vi "Finish.vi"   [LabVIEW 2015]
doc: "This VI is called just before exiting. It is expected to close I/O refnum, save collected data, etc."
uses:
  <vilib>/Rock Robotics/WPI/Utilities/WPI_GetSetVariantRefNum.vi
  <vilib>/Rock Robotics/WPI/Ultrasonic/WPI_SonarMB1010DigitalRefNum Registry Get.vi
  <vilib>/Rock Robotics/WPI/Ultrasonic/WPI_SonarMB1010DigitalClose.vi
types:
  T1 = typedef "WPI_SonarMB1010DigitalDeviceRef.ctl" = cluster{"CounterDevRef":T2, "Scaling factor (s/in)":dbl}
  T2 = typedef "WPI_CounterDevRef.ctl" = cluster{"DevStatus":errorcluster, "CntIndex":T3}
  T3 = typedef "FPGA_CounterCtrSystemIndex.ctl" = enum8{"Ctr 0", "Ctr 1", "Ctr 2", "Ctr 3", "Ctr 4", "Ctr 5", "Ctr 6", "Ctr 7", "Invalid"}
  T4 = typedef "WPI_JoystickDevRef.ctl" = cluster{"Device":T5}
  T5 = typedef "WPI_JoystickDeviceEnum.ctl" = enum16{"USB 0", "USB 1", "USB 2", "USB 3", "USB 4", "USB 5"}
  T6 = typedef "WPI_MotorControlDeviceRef.ctl" = cluster{"DeviceStatus":errorcluster, "Type":T7, "PWM":cluster{"PWM Channel":T8, "DeadBand":T9}, "CAN":cluster{"Device Number":u8, "Control Mode":T10, "Semaphore":T11, "Max Vout":dbl, "TalonSRX Control Mode":T12}, "Invert":bool}
  T7 = typedef "WPI_MotorControlType.ctl" = enum16{"PWM", "CAN", "CANTalonSRX"}
  T8 = typedef "FPGA_DIOPWMChannel.ctl" = enum8{"PWM 0", "PWM 1", "PWM 2", "PWM 3", "PWM 4", "PWM 5", "PWM 6", "PWM 7", "PWM 8", "PWM 9", "PWM MXP 0", "PWM MXP 1", "PWM MXP 2", "PWM MXP 3", "PWM MXP 4", "PWM MXP 5", "PWM MXP 6", "PWM MXP 7", "PWM MXP 8", "PWM MXP 9", "Invalid"}
  T9 = typedef "WPI_PWMDeadband.ctl" = cluster{"Name":string, "maxPositivePwm":i32, "minPositivePwm":i32, "centerPwm":i32, "maxNegativePwm":i32, "minNegativePwm":i32, "angularRange":u16}
  T10 = typedef "WPI_CANJaguar_ControlMode.ctl" = enum8{"Percent VBus", "Current", "Speed", "Position", "Voltage"}
  T11 = typedef "Semaphore RefNum" = refnum<k1>
  T12 = typedef "WPI_CANTalonSRX_APIControlMode.ctl" = enum8{"Percent VBus", "Speed", "Position", "Slave", "Unchanged / Invalid", "Voltage Compensation", "Current", "Motion Profile"}
  T13 = typedef "WPI_ServoDeviceRef.ctl" = cluster{"DeviceStatus":errorcluster, "PWM Channel":T8, "DeadBand":T9}
  T14 = typedef "WPI_AccelerometerDevRef.ctl" = cluster{"DevStatus":errorcluster, "Scaling":T15, "Analog Channels":T16, "I2C Bus":T18, "SPI Bus":T19, "Accel Range":T20, "ADXL Axes":T21, "Handle":i32, "Device Address":u8, "Accel Type":enum16{"Analog", "ADXL345 I2C", "ADXL345 SPI", "Internal", "ADXL362 SPI"}}
  T15 = typedef "WPI_AccelerometerScaling.ctl" = cluster{"Gain (VoltsPerG)":dbl, "Center Voltage":dbl}
  T16 = typedef "WPI_AccelerometerAnalogChannels.ctl" = cluster{"X-Axis":T17, "Y-Axis":T17, "Z-Axis":T17}
  T17 = typedef "FPGA_AIChannel.ctl" = enum8{"AI 0", "AI 1", "AI 2", "AI 3", "AI MXP 0", "AI MXP 1", "AI MXP 2", "AI MXP 3", "Invalid"}
  T18 = typedef "i2c_bus.ctl" = enum16{"I2C On-Board", "I2C MXP", "Invalid"}
  T19 = typedef "spi_bus.ctl" = enum16{"SPI On-Board, CS0", "SPI On-Board, CS1", "SPI On-Board, CS2", "SPI On-Board, CS3", "SPI MXP", "Invalid"}
  T20 = typedef "ADXL345 Range.ctl" = u8
  T21 = typedef "WPI_AccelerometerADXL345 Axes.ctl" = cluster{"X-Axis":bool, "Y-Axis":bool, "Z-Axis":bool}
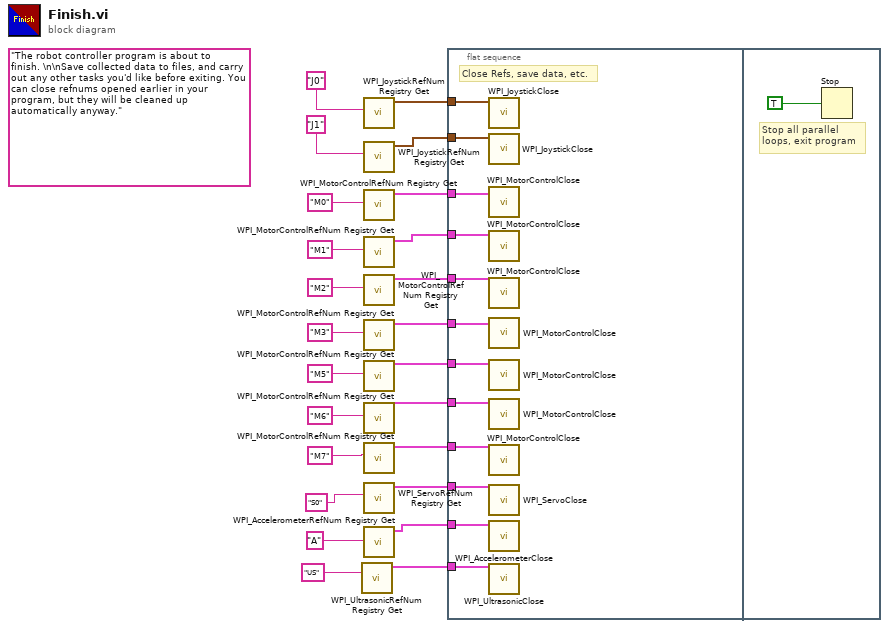
[diagram p0: block diagram]
diagram:
  (unwired) "The robot controller program is about to finish. \n\nSave collected data to files, and carry out any other tasks you'd like before exiting. You can close refnums opened earlier in your program, but they will be cleaned up automatically anyway."
  n1 = call-poly <vilib>:"WPI_UltrasonicRefNum Registry Get.vi"("refnum name"="US") -> ("SonarMB1010DigitalDevRef"=w2:T1)  [unwired: 9 in, 1 out]
  n2 = call <vilib>:"WPI_JoystickRefNum Registry Get.vi"("refnum name"="J0") -> ("JoystickDevRef"=w23:T4)  [unwired: 1 in, 9 out]
  n3 = call <vilib>:"WPI_JoystickRefNum Registry Get.vi"("refnum name"="J1") -> ("JoystickDevRef"=w21:T4)  [unwired: 1 in, 9 out]
  n4 = call <vilib>:"WPI_MotorControlRefNum Registry Get.vi"("refnum name"="M0") -> ("MotorControlDevRef"=w20:T6)  [unwired: 9 in, 1 out]
  n5 = call <vilib>:"WPI_MotorControlRefNum Registry Get.vi"("refnum name"="M1") -> ("MotorControlDevRef"=w13:T6)  [unwired: 9 in, 1 out]
  n6 = call <vilib>:"WPI_MotorControlRefNum Registry Get.vi"("refnum name"="M2") -> ("MotorControlDevRef"=w12:T6)  [unwired: 9 in, 1 out]
  n7 = call <vilib>:"WPI_MotorControlRefNum Registry Get.vi"("refnum name"="M3") -> ("MotorControlDevRef"=w11:T6)  [unwired: 9 in, 1 out]
  n8 = call <vilib>:"WPI_MotorControlRefNum Registry Get.vi"("refnum name"="M5") -> ("MotorControlDevRef"=w10:T6)  [unwired: 9 in, 1 out]
  n9 = call <vilib>:"WPI_MotorControlRefNum Registry Get.vi"("refnum name"="M6") -> ("MotorControlDevRef"=w9:T6)  [unwired: 9 in, 1 out]
  n10 = call <vilib>:"WPI_MotorControlRefNum Registry Get.vi"("refnum name"="M7") -> ("MotorControlDevRef"=w7:T6)  [unwired: 9 in, 1 out]
  n11 = call <vilib>:"WPI_ServoRefNum Registry Get.vi"("refnum name"="S0") -> ("ServoDeviceRef"=w6:T13)  [unwired: 9 in, 1 out]
  n12 = call <vilib>:"WPI_AccelerometerRefNum Registry Get.vi"("refnum name"="A") -> ("AccelerometerDevRef"=w4:T14)  [unwired: 9 in, 1 out]
  n13 = flat-sequence {
    tunnel: w23 -> [w36]
    tunnel: w21 -> [w35]
    tunnel: w20 -> [w34]
    tunnel: w13 -> [w33]
    tunnel: w12 -> [w32]
    tunnel: w11 -> [w31]
    tunnel: w10 -> [w30]
    tunnel: w9 -> [w29]
    tunnel: w7 -> [w28]
    tunnel: w6 -> [w27]
    tunnel: w4 -> [w26]
    tunnel: w2 -> [w25]
    frame #0 {
      # "Close Refs, save data, etc."
      n14 = call <vilib>:"WPI_JoystickClose.vi"("JoystickDevRef"=w36) -> ()  [unwired: 11 out]
      n15 = call <vilib>:"WPI_JoystickClose.vi"("JoystickDevRef"=w35) -> ()  [unwired: 11 out]
      n16 = call <vilib>:"WPI_MotorControlClose.vi"("MotorControlDevRef"=w34) -> ()  [unwired: 10 in, 1 out]
      n17 = call <vilib>:"WPI_MotorControlClose.vi"("MotorControlDevRef"=w33) -> ()  [unwired: 10 in, 1 out]
      n18 = call <vilib>:"WPI_MotorControlClose.vi"("MotorControlDevRef"=w32) -> ()  [unwired: 10 in, 1 out]
      n19 = call <vilib>:"WPI_MotorControlClose.vi"("MotorControlDevRef"=w31) -> ()  [unwired: 10 in, 1 out]
      n20 = call <vilib>:"WPI_MotorControlClose.vi"("MotorControlDevRef"=w30) -> ()  [unwired: 10 in, 1 out]
      n21 = call <vilib>:"WPI_MotorControlClose.vi"("MotorControlDevRef"=w29) -> ()  [unwired: 10 in, 1 out]
      n22 = call <vilib>:"WPI_MotorControlClose.vi"("MotorControlDevRef"=w28) -> ()  [unwired: 10 in, 1 out]
      n23 = call <vilib>:"WPI_ServoClose.vi"("ServoDeviceRef"=w27) -> ()  [unwired: 10 in, 1 out]
      n24 = call <vilib>:"WPI_AccelerometerClose.vi"("AccelerometerDevRef"=w26) -> ()  [unwired: 10 in, 1 out]
      n25 = call-poly <vilib>:"WPI_UltrasonicClose.vi"("SonarMB1010DigitalDevRef"=w25) -> ()  [unwired: 10 in, 1 out]
    }
    frame #1 {
      # "Stop all parallel\nloops, exit program"
      n26 = Stop(stop? (T)=TRUE ("Quit")) -> ()
    }
  }
